vi "Dequeue Message.vi"(8 "error in (no error)":errorcluster, 11 "Queue in":refnum<queue>) -> (0 "error out":errorcluster, 2 "Message":string, 3 "Queue Out":refnum<queue>)   [LabVIEW 2024, in "View.lvlib"]
uses:
  View.lvlib
  Type Defs/QMH Message--cluster.ctl
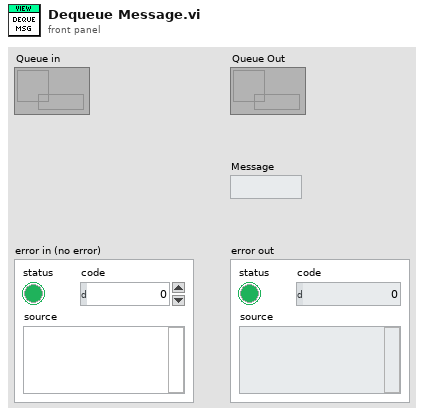
[diagram p1: front panel]
types:
  T1 = typedef "View.lvlib/QMH Message--cluster.ctl" = cluster{"Message":string, "Message Data":variant}
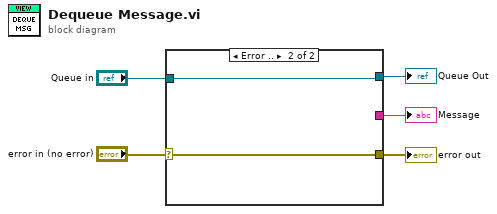
[diagram p0: block diagram]
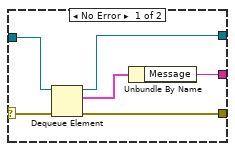
[diagram p2: hidden frame]
diagram:
  n1 = case shown="Error .." "error in (no error)" {
    selector: "error in (no error)" -> [w10 w12]
    tunnel: "Queue in" -> [w9 w13]
    tunnel: [w8 w12] -> w3
    tunnel: [w7 w13] -> w2
    tunnel: [w6 _] -> w1
    frame No Error {
      n2 = Dequeue Element(queue=w9, error in (no error)=w10) -> (queue out=w7:refnum<queue>, element=w11:T1, error out=w8:errorcluster)  [unwired: 1 in, 1 out]
      n3 = Unbundle By Name(w11) -> ("Message"=w6:string)
    }
    frame Error {
    }
  }
  "error out" <- w3
  "Queue Out" <- w2
  "Message" <- w1
